vi "读写.vi"(0 "TCP Connection Ref":refnum<k5>, 1 "Read / Write":u8(ring)=4 items=["Read"=4, "Write"=5], 2 "Address Areas":u8(ring)=131 items=["I/O (P)"=128, "Input (I)"=129, "Output (Q)"=130, "Bit Memory (M)"=131, "Data (DB)"=132, "Instance Data (DI)"=133, "Local Data (L)"=134, "Predecessor Local Data (VL)"=135], 3 "Start Address (bytes)":u32, 4 "Data Block #":u16=1, 5 "Read Length (bytes)":u16=1, 6 "Write Data":i32, 7 "error in":errorcluster) -> (20 "TCP Connection Ref Out":refnum<k5>, 22 "Read Data":u8[](array[numeric]) format="%.0x", 24 "Data Element 0 as Boolean array":bool[](array[boolean]), 26 "Data Valid":bool, 27 "error out":errorcluster)   [LabVIEW 2017]
uses:
  S7 TCP API Library/S7 TCP.lvlib
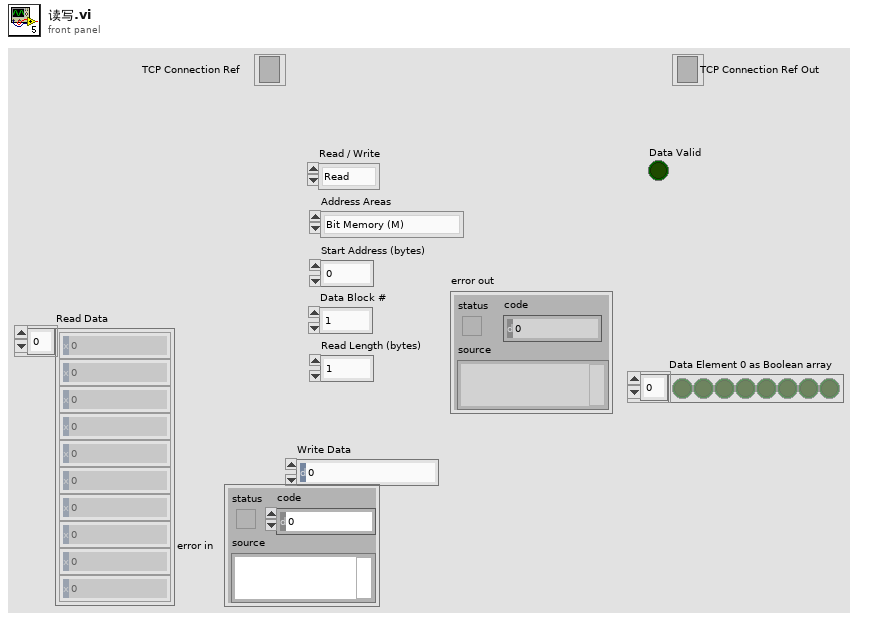
[diagram p1: front panel]
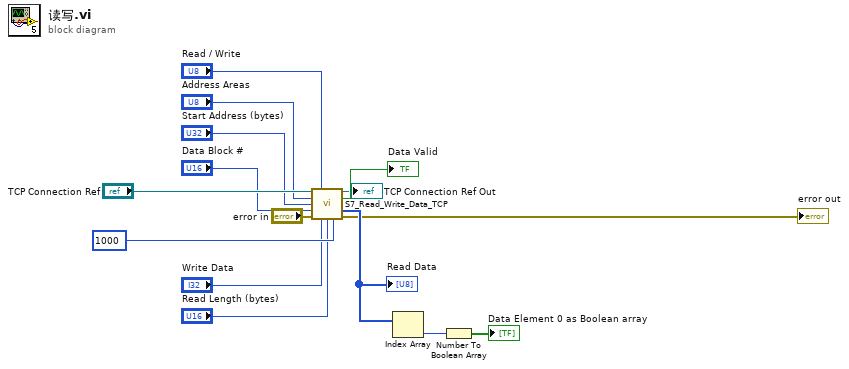
[diagram p0: block diagram]
diagram:
  n1 = call "S7_Read_Write_Data_TCP.vi"("TCP Connection Ref"="TCP Connection Ref", "Read / Write"="Read / Write", "Address Areas"="Address Areas", "Start Address (bytes)"="Start Address (bytes)", "Data Block #"="Data Block #", "error in"="error in", "Write Data"="Write Data", "Length (bytes)"="Read Length (bytes)", "Timeout"=u32 1000 ("Request Timeout")) -> ("TCP Connection Ref Out"=→"TCP Connection Ref Out":refnum<k5>, "Data Valid"=→"Data Valid":bool, "Data Read"=w8:u8[], "error out"=→"error out":errorcluster)  [unwired: 1 in, 2 out]
  "Read Data" <- w8
  n2 = Index Array(array=w8) -> (element=w7:u8)  [unwired: 1 in]
  n3 = Number To Boolean Array(number=w7) -> (Boolean array=→"Data Element 0 as Boolean array":bool[])
